vi "ConfigurationBooltoString.vi"(10 "TriggerMode":bool, 11 "MeasurementMode":bool) -> (2 "OutString":string)   [LabVIEW 2020]
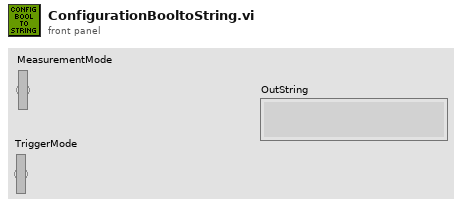
[diagram p1: front panel]
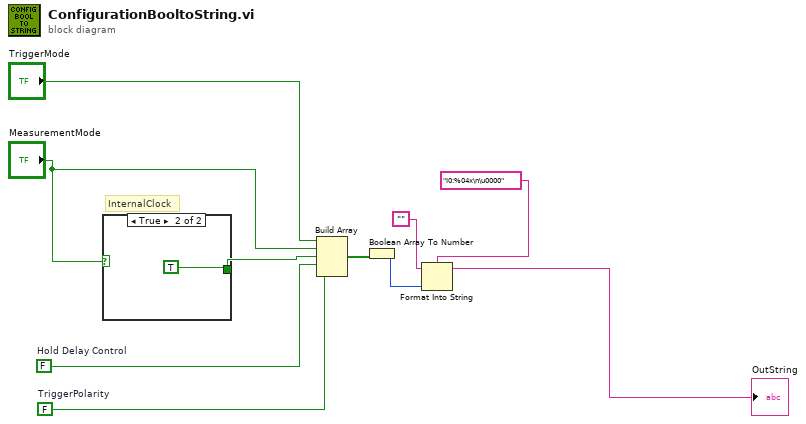
[diagram p0: block diagram]
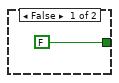
[diagram p2: hidden frame]
diagram:
  w4 = FALSE  # TriggerPolarity
  w5 = FALSE  # Hold Delay Control
  # "InternalClock"
  n1 = case shown="True" "MeasurementMode" {
    tunnel: [FALSE TRUE] -> w6
    frame False {
    }
    frame True {
    }
  }
  n2 = Build Array("TriggerMode", "MeasurementMode", w6, w5, w4) -> (w9:bool[])
  n3 = Boolean Array To Number(Boolean array=w9) -> (number=w10:u32)
  n4 = Format Into String(format string="I0:%04x\n\u0000" ("chaîne de format"), initial string="", w10) -> (resulting string=→"OutString":string)  [unwired: 1 in, 1 out]
